vi "Global.vi"() -> ()   [LabVIEW 2019, in "Memory Data Access.lvlib"]
uses:
  Memory Data Access.lvlib
panel:
  in  "MAX_STR_LEN":i32=1024
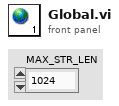
[diagram p1: front panel]
diagram:
